vi "FGV_Start-Live.vi"(8 "error in":errorcluster, 10 "Action":T1, 11 "Start/Live (0/1) IN":bool) -> (0 "error out":errorcluster, 3 "Start/Live (0/1) OUT":bool)   [LabVIEW 2026]
doc: "Functional Global Variable:\n- Write the value into the memory \nor\n- Read the value from the memory"
uses:
  TypeDef_FGV.ctl
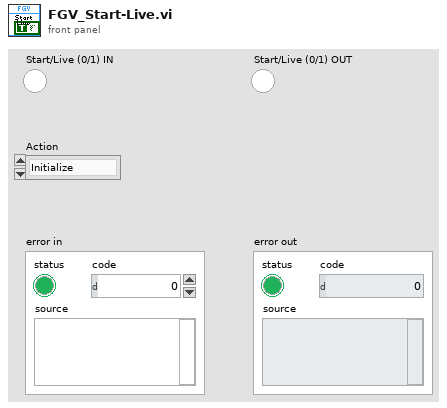
[diagram p1: front panel]
types:
  T1 = typedef "TypeDef_FGV.ctl" = enum16{"Initialize", "Write", "Read", "Read_File", "Write_to_File"}
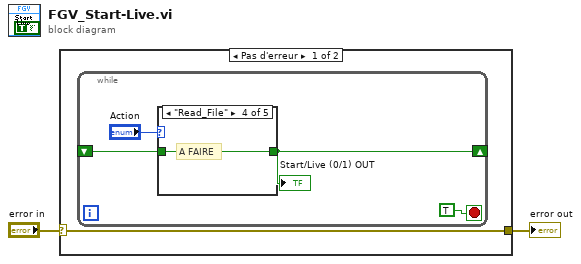
[diagram p0: block diagram]
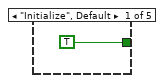
[diagram p2: hidden frame]
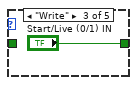
[diagram p4: hidden frame]
diagram:
  n1 = case shown="Pas d'erreur" "error in" {
    selector: "error in" -> [w3 w13]
    tunnel: [w3 w13] -> w1
    frame No Error {
      n2 = while {
        shift-right: [w4] -> _
        shift-left: _ -> [w5]
        stop <- TRUE stop-if-true
        n3 = case shown="\"Read_File\"" "Action" {
          tunnel: w5 -> [_ w9 _ w11 w12]
          tunnel: [TRUE w9 "Start/Live (0/1) IN" w11 w12] -> w4
          frame "Initialize", Default {
          }
          frame "Read" {
          }
          frame "Write" {
          }
          frame "Read_File" {
            # "A FAIRE"
          }
          frame "Write_to_File" {
            # "A Faire"
          }
        }
        "Start/Live (0/1) OUT" <- w4
      }
    }
    frame Error {
    }
  }
  "error out" <- w1
